vi "Grid Animation.vi"() -> ()   [LabVIEW 2026]
uses:
  <vilib>/FPGAPlugInAG/cRIO-9047/niLvFpga_Open_cRIO-9047.vi
  <vilib>/rvi/interface/common/dynamic/niFpgaDynamicAddResources.vi
  <vilib>/FPGAPlugInAG/Dynamic/niLvFpga_Run_Dynamic.vi
  <vilib>/rvi/interface/common/dynamic/niFpgaDynamicGetExecutionMode.vi
  <vilib>/Utility/error.llb/Error Cluster From Error Code.vi
  <vilib>/rvi/errors/niLvFpgaAdjustHostInterfaceError.vi
  <vilib>/FPGAPlugInAG/Dynamic/niLvFpga_Abort_Dynamic.vi
  <vilib>/FPGAPlugInAG/Dynamic/niLvFpga_Close_Dynamic.vi
  <vilib>/rvi/interface/nirviOpenFPGA/nirviOpenFPGA.xnode
  Speed of VIght/FPGA Bitfiles/speedofvight_FPGATarget_PWMTest_tivD2XU7OY8.lvbitx
  Speed of VIght/PWM Test.vi
  <vilib>/rvi/interface/nirviMethod/nirviMethod.xnode
  <vilib>/FPGA/interface/niFpgaViExecutionMode.ctl
  <vilib>/rvi/interface/nirviReadWriteControl/nirviReadWriteControl.xnode
  <vilib>/rvi/interface/nirviCloseFPGA/nirviCloseFPGA.xnode
  NiFpgaLv.dll
  <vilib>/rvi/interface/Simulation/niFpgaSimulationCallBeginRW.vi
panel:
  in  "Period":u16
  in  "Horizontal Pointer Slide":dbl(slide) scale=0.0..1.0
  in  "Effect":T1(ring)
  out "2D Picture":picture
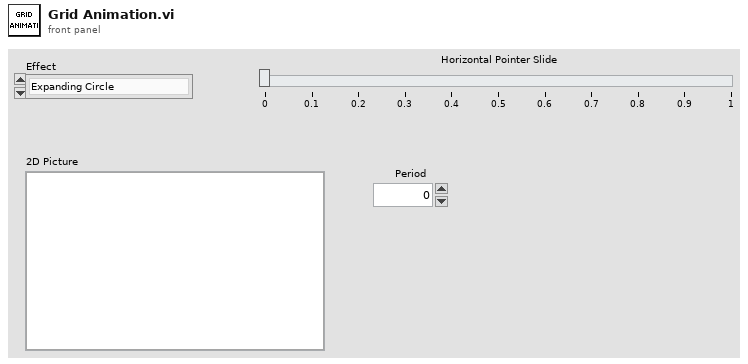
[diagram p1: front panel]
types:
  T1 = enum16{"Expanding Circle", "Plasma", "Radar Sweep", "Matrix Rain", "Campfire", "Diagonal Scan"}
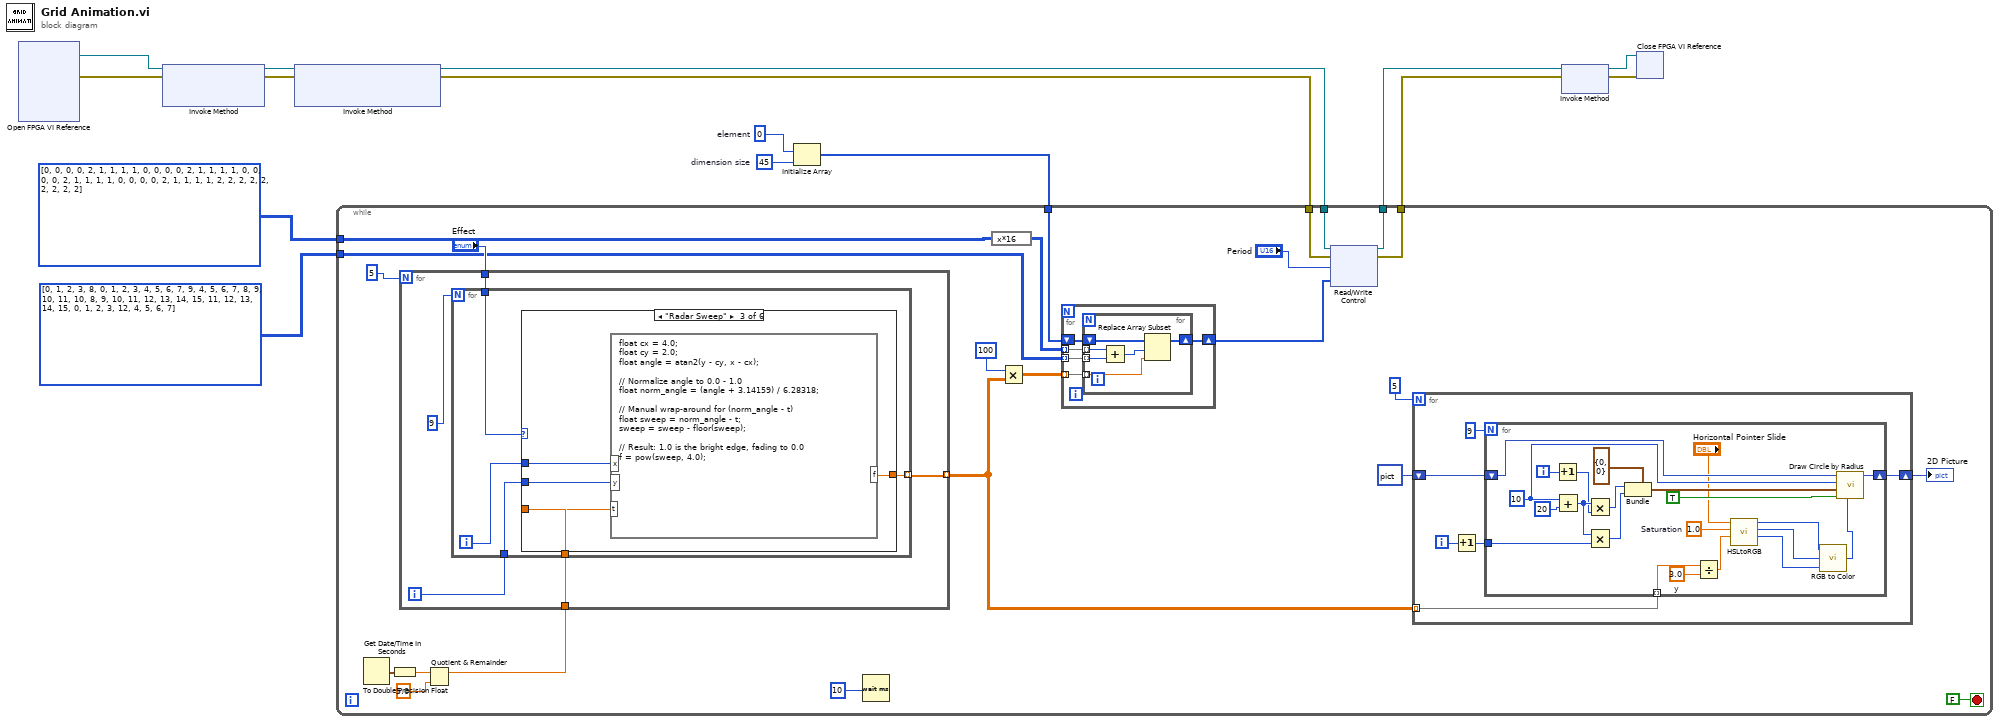
[diagram p0: block diagram]
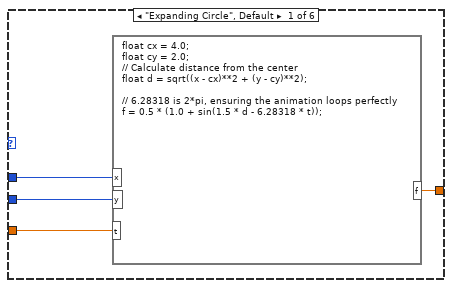
[diagram p2: hidden frame]
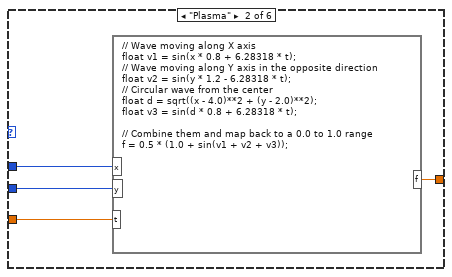
[diagram p3: hidden frame]
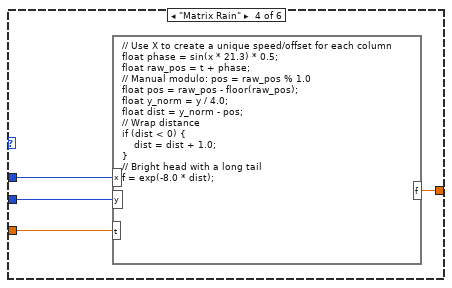
[diagram p4: hidden frame]
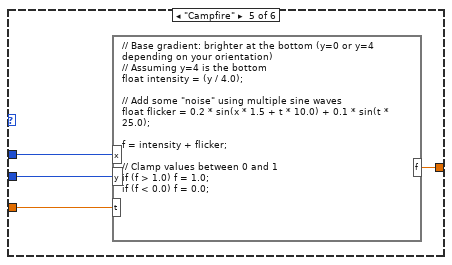
[diagram p5: hidden frame]
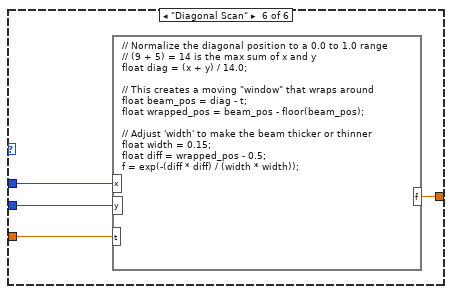
[diagram p6: hidden frame]
diagram:
  w4 = u16 0  # element
  w5 = 45  # dimension size
  n1 = xnode "Open FPGA VI Reference"() -> ("FPGA VI Reference Out"=w10:refnum<k20>, "error out"=w11:errorcluster)  [unwired: 2 in]
  n2 = xnode "Invoke Method"("FPGA VI Reference In"=w10, "error in"=w11) -> ("FPGA VI Reference Out"=w12:refnum<k20>, "error out"=w13:errorcluster)  [unwired: 1 in]
  n3 = xnode "Invoke Method"("FPGA VI Reference In"=w12, "error in"=w13) -> ("FPGA VI Reference Out"=w9:refnum<k20>, "error out"=w8:errorcluster)  [unwired: 1 out]
  n4 = Initialize Array(w4, w5) -> (w3:u16[])
  n5 = while {
    tunnel: w9 -> [w28]
    tunnel: w8 -> [w27]
    tunnel: [w26] -> w7
    tunnel: [w25] -> w6
    tunnel: w3 -> [w23]
    tunnel: i32[][] [[0, 0, 0, 0, 2, 1, 1, 1, 1], [0, 0, 0, 0, 2, 1, 1, 1, 1], [0, 0, 0, 0, 2, 1, 1, 1, 1], [0, 0, 0, 0, 2, 1, 1, 1, 1], [2, 2, 2, 2, 2, 2, 2, 2, 2]] -> [w20]
    tunnel: i32[][] [[0, 1, 2, 3, 8, 0, 1, 2, 3], [4, 5, 6, 7, 9, 4, 5, 6, 7], [8, 9, 10, 11, 10, 8, 9, 10, 11], [12, 13, 14, 15, 11, 12, 13, 14, 15], [0, 1, 2, 3, 12, 4, 5, 6, 7]] -> [w18]
    stop <- FALSE stop-if-true
    n6 = Get Date/Time In Seconds() -> (seconds since 1Jan1904=w36:timestamp)
    n7 = To Double Precision Float(number=w36) -> (double precision float=w35:dbl)
    n8 = Quotient & Remainder(x=w35, y=5.0) -> (x-y*floor(x/y)=w33:dbl)  [unwired: 1 out]
    n9 = for {
      N: 5 -> [_]
      tunnel: w33 -> [w53]
      tunnel: [w52] -> w24 mode=indexing
      tunnel: "Effect" -> [w51]
      i -> [w54]
      n10 = for {
        N: 9 -> [_]
        tunnel: w54 -> [w59]
        tunnel: w53 -> [w58]
        tunnel: [w57] -> w52 mode=indexing
        tunnel: w51 -> [w56]
        i -> [w60]
        n11 = case shown="\"Radar Sweep\"" w56 {
          tunnel: w60 -> [w64 w68 w72 w76 w80 w84]
          tunnel: w59 -> [w63 w67 w71 w75 w79 w83]
          tunnel: w58 -> [w62 w66 w70 w74 w78 w82]
          tunnel: [w61 w65 w69 w73 w77 w81] -> w57
          frame "Expanding Circle", Default {
            n12 = formula code="float cx = 4.0;\nfloat cy = 2.0;\n// Calculate distance from the center\nfloat d = sqrt((x - cx)**2 + (y - cy)**2);\n\n// 6.28318 is 2*pi, ensuring the animation loops perfectly\nf = 0.5 * (1.0 + sin(1.5 * d - 6.28318 * t));"("x"=w64, "y"=w63, "t"=w62) -> ("f"=w61:dbl)
          }
          frame "Plasma" {
            n13 = formula code="// Wave moving along X axis\nfloat v1 = sin(x * 0.8 + 6.28318 * t);\n// Wave moving along Y axis in the opposite direction\nfloat v2 = sin(y * 1.2 - 6.28318 * t);\n// Circular wave from the center\nfloat d = sqrt((x - 4.0)**2 + (y - 2.0)**2);\nfloat v3 = sin(d * 0.8 + 6.28318 * t);\n\n// Combine them and map back to a 0.0 to 1.0 range\nf = 0.5 * (1.0 + sin(v1 + v2 + v3));"("x"=w68, "y"=w67, "t"=w66) -> ("f"=w65:dbl)
          }
          frame "Radar Sweep" {
            n14 = formula code="float cx = 4.0;\nfloat cy = 2.0;\nfloat angle = atan2(y - cy, x - cx);\n\n// Normalize angle to 0.0 - 1.0\nfloat norm_angle = (angle + 3.14159) / 6.28318;\n\n// Manual wrap-around for (norm_angle - t)\nfloat sweep = norm_angle - t;\nsweep = sweep - floor(sweep); \n\n// Result: 1.0 is the bright edge, fading to 0.0\nf = pow(sweep, 4.0);"("x"=w72, "y"=w71, "t"=w70) -> ("f"=w69:dbl)
          }
          frame "Matrix Rain" {
            n15 = formula code="// Use X to create a unique speed/offset for each column\nfloat phase = sin(x * 21.3) * 0.5; \nfloat raw_pos = t + phase;\n// Manual modulo: pos = raw_pos % 1.0\nfloat pos = raw_pos - floor(raw_pos);\nfloat y_norm = y / 4.0;\nfloat dist = y_norm - pos;\n// Wrap distance\nif (dist < 0) {\n    dist = dist + 1.0;\n}\n// Bright head with a long tail\nf = exp(-8.0 * dist);"("x"=w76, "y"=w75, "t"=w74) -> ("f"=w73:dbl)
          }
          frame "Campfire" {
            n16 = formula code="// Base gradient: brighter at the bottom (y=0 or y=4 depending on your orientation)\n// Assuming y=4 is the bottom\nfloat intensity = (y / 4.0);\n\n// Add some \"noise\" using multiple sine waves\nfloat flicker = 0.2 * sin(x * 1.5 + t * 10.0) + 0.1 * sin(t * 25.0);\n\nf = intensity + flicker;\n\n// Clamp values between 0 and 1\nif (f > 1.0) f = 1.0;\nif (f < 0.0) f = 0.0;"("x"=w80, "y"=w79, "t"=w78) -> ("f"=w77:dbl)
          }
          frame "Diagonal Scan" {
            n17 = formula code="// Normalize the diagonal position to a 0.0 to 1.0 range\n// (9 + 5) = 14 is the max sum of x and y\nfloat diag = (x + y) / 14.0; \n\n// This creates a moving \"window\" that wraps around\nfloat beam_pos = diag - t;\nfloat wrapped_pos = beam_pos - floor(beam_pos);\n\n// Adjust 'width' to make the beam thicker or thinner\nfloat width = 0.15;\nfloat diff = wrapped_pos - 0.5;\nf = exp(-(diff * diff) / (width * width));"("x"=w84, "y"=w83, "t"=w82) -> ("f"=w81:dbl)
          }
        }
      }
    }
    n18 = Wait (ms)(milliseconds to wait=u32 10) -> ()  [unwired: 1 out]
    n19 = expression code="x*16"(w20) -> (w19:i32[][])
    n20 = Multiply(x=100, y=w24) -> (x*y=w22:dbl[][])
    n21 = for {
      shift-right: [w43] -> w17
      shift-left: w23 -> [w44]
      tunnel: w22 -> [w42] mode=indexing
      tunnel: w19 -> [w41] mode=indexing
      tunnel: w18 -> [w40] mode=indexing
      n22 = for {
        shift-right: [w49] -> w43
        shift-left: w44 -> [w50]
        tunnel: w42 -> [w48] mode=indexing
        tunnel: w41 -> [w47] mode=indexing
        tunnel: w40 -> [w46] mode=indexing
        n23 = Add(x=w47, y=w46) -> (x+y=w45:i32)
        n24 = Replace Array Subset(array=w50, new element=w48, index=w45) -> (w49:u16[])
      }
    }
    n25 = xnode "Read/Write Control"("FPGA VI Reference In"=w28, "error in"=w27, "Period"="Period", "x"=w17) -> ("FPGA VI Reference Out"=w26:refnum<k20>, "error out"=w25:errorcluster)
    n26 = for {
      N: 5 -> [_]
      shift-right: [w90] -> w38
      shift-left: picture data[5B] ("new picture") -> [w89]
      tunnel: w24 -> [w85] mode=indexing
      i -> [w88]
      n27 = Increment(x=w88) -> (x+1=w86:i32)
      n28 = for {
        N: 9 -> [_]
        shift-right: [w112] -> w90
        shift-left: w89 -> [w111]
        tunnel: w86 -> [w106]
        tunnel: w85 -> [w93] mode=indexing
        i -> [w108]
        w92 = 3.0  # y
        w97 = 1.0  # Saturation
        w110 = i16 10 ("radius")
        n29 = Increment(x=w108) -> (x+1=w100:i32)
        n30 = Add(x=w110, y=i16 20 ("radius")) -> (x+y=w107:i16)
        n31 = Multiply(x=w107, y=w100) -> (x*y=w103:i32)
        n32 = Multiply(x=w107, y=w106) -> (x*y=w102:i32)
        n33 = Bundle(cluster=cluster{"horizontal":i16, "vertical":i16} {"horizontal"=0, "vertical"=0} ("pixel center"), "horizontal"=w103, "vertical"=w102) -> (w104:cluster{"horizontal":i16, "vertical":i16})
        n34 = Divide(x=w93, y=w92) -> (x/y=w91:dbl)
        n35 = call "HSLtoRGB.vi"("Lightness"=w91, "Saturation"=w97, "Hue"="Horizontal Pointer Slide") -> ("Blue"=w95:u8, "Green"=w94:u8, "Red"=w96:u8)  [unwired: 6 in]
        n36 = call <vilib>:"RGB to Color.vi"("B"=w95, "G"=w94, "R"=w96) -> ("Color"=w99:u32)
        n37 = call <vilib>:"Draw Circle by Radius.vi"("color(black)"=w99, "fill?(F)"=TRUE, "pixel center"=w104, "radius"=w110, "picture"=w111) -> ("new picture"=w112:picture)  [unwired: 6 in]
      }
    }
    "2D Picture" <- w38
  }
  n38 = xnode "Invoke Method"("FPGA VI Reference In"=w7, "error in"=w6) -> ("FPGA VI Reference Out"=w14:refnum<k20>, "error out"=w15:errorcluster)
  n39 = xnode "Close FPGA VI Reference"("FPGA VI Reference In"=w14, "error in"=w15) -> ()  [unwired: 1 out]
